vi "record_pol_value.vi"(7 "file_base_name":string="polarization", 8 "value":dbl format="%#_13g", 11 "date_time":timestamp) -> ()   [LabVIEW 2019]
uses:
  <vilib>/Utility/file.llb/Write Delimited Spreadsheet (string).vi
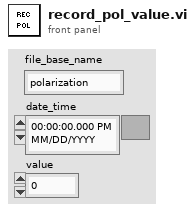
[diagram p1: front panel]
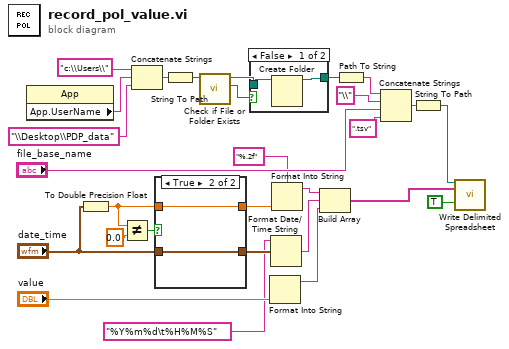
[diagram p0: block diagram]
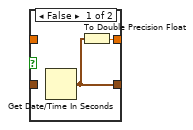
[diagram p2: hidden frame]
diagram:
  n1 = property class="App"() -> ("App.UserName"=w25:string)  [unwired: 2 in, 2 out]
  n2 = To Double Precision Float(number="date_time") -> (double precision float=w5:dbl)
  n3 = Not Equal?(x=w5, y=0.0) -> (x != y?=w11:bool)
  n4 = Concatenate Strings("c:\\Users\\", w25, "\\Desktop\\PDP_data") -> (w23:string)
  n5 = case shown="True" w11 {
    tunnel: [w29 w32] -> w3
    tunnel: "date_time" -> [_ w32]
    tunnel: [w30 w31] -> w6
    tunnel: w5 -> [_ w31]
    frame False {
      n6 = Get Date/Time In Seconds() -> (seconds since 1Jan1904=w29:timestamp)
      n7 = To Double Precision Float(number=w29) -> (double precision float=w30:dbl)
    }
    frame True {
    }
  }
  n8 = String To Path(string=w23) -> (path=w18:path)
  n9 = call <vilib>:"Check if File or Folder Exists.vi"("path"=w18) -> ("file or folder exists?"=w17:bool, "dup path"=w15:path)  [unwired: 8 in, 1 out]
  n10 = case shown="False" w17 {
    tunnel: w15 -> [w34 w35]
    tunnel: [w33 w35] -> w16
    frame False {
      n11 = Create Folder(path (use dialog)=w34) -> (created path=w33:path)  [unwired: 2 in, 2 out]
    }
    frame True {
    }
  }
  n12 = Format Into String("value") -> (resulting string=w7:string)  [unwired: 3 in, 1 out]
  n13 = Format Date/Time String(time format string (%c)="%Y%m%d\t%H%M%S" ("format string"), seconds (now)=w3) -> (date/time string=w4:string)  [unwired: 1 in]
  n14 = Format Into String(format string="%.2f", w6) -> (resulting string=w8:string)  [unwired: 2 in, 1 out]
  n15 = Build Array(w8, w4, w7) -> (w28:string[])
  n16 = Path To String(path=w16) -> (string=w14:string)
  n17 = Concatenate Strings(w14, "\\", "file_base_name", ".tsv" ("string")) -> (w19:string)
  n18 = String To Path(string=w19) -> (path=w13:path)
  n19 = call-poly <vilib>:"Write Delimited Spreadsheet.vi"("file path (dialog if empty)"=w13, "1D data"=w28, "append to file? (new file:F)"=TRUE) -> ()  [unwired: 11 in, 2 out]
